vi "DLTS - reset bias (SubVI).vi"(8 "error in (no error)":errorcluster, 11 "Handle in":T1 {"Handle" format="0x%08x"; "Conn" format="0x%08x"}) -> (0 "error out":errorcluster, 3 "Handle out":T1 {"Handle" format="0x%08x"; "Conn" format="0x%08x"})   [LabVIEW 2019]
doc: "Resets bias voltage after DLTS measurement"
uses:
  <instrlib>/Zurich Instruments LabOne/Public/ziTypeHandle.ctl
  <instrlib>/Zurich Instruments LabOne/Public/Configure/ziSetValueDoubleArray.vi
  <instrlib>/Zurich Instruments LabOne/Zurich Instruments LabOne.lvlib
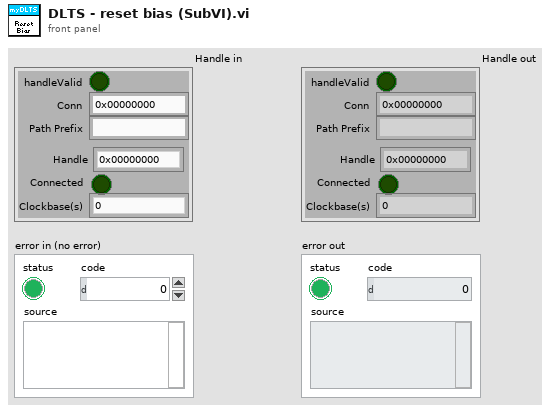
[diagram p1: front panel]
types:
  T1 = typedef "Zurich Instruments LabOne.lvlib/ziTypeHandle.ctl" = cluster{"handleValid":bool, "Conn":u64, "Path Prefix":string, "Handle":u64, "Connected":bool, "Clockbase(s)":dbl}
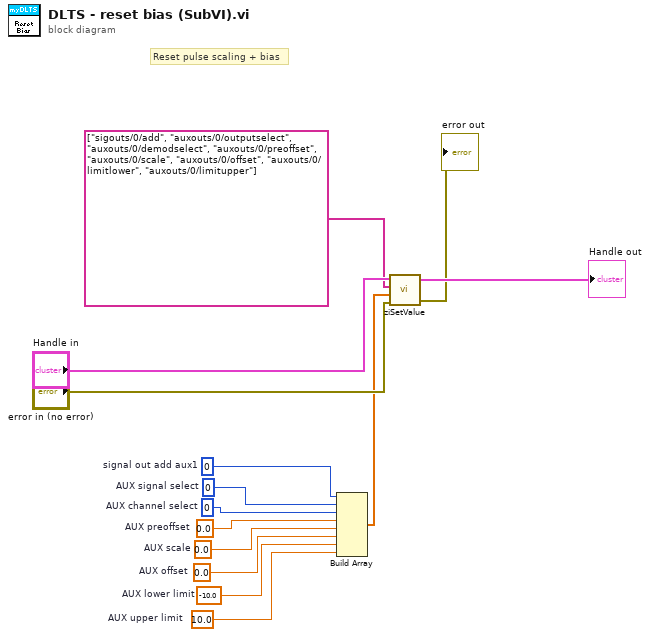
[diagram p0: block diagram]
diagram:
  w1 = 0  # signal out add aux1
  w8 = 10.0  # AUX upper limit
  w7 = -10.0  # AUX lower limit
  w6 = 0.0  # AUX offset
  w5 = 0.0  # AUX scale
  w4 = 0.0  # AUX preoffset
  w3 = 0  # AUX channel select
  w2 = 0  # AUX signal select
  # "Reset pulse scaling + bias"
  n1 = Build Array(w1, w2, w3, w4, w5, w6, w7, w8) -> (w10:dbl[])
  n2 = call-poly <instrlib>:"ziSetValue.vi"("Error In"="error in (no error)", "Values"=w10, "Paths"=string[] ["sigouts/0/add", "auxouts/0/outputselect", "auxouts/0/demodselect", "auxouts/0/preoffset", "auxouts/0/scale", "auxouts/0/offset", "auxouts/0/limitlower", "auxouts/0/limitupper"], "Handle In"="Handle in") -> ("Error Out"=→"error out":errorcluster, "Handle Out"=→"Handle out":T1)  [unwired: 1 in]
